vi "Configure Library Classes in Memory for Build.vi"(5 "skip inline classes":string[](array[string]), 7 "target name (My Computer)":string="My Computer", 10 "save VIs? (T)":bool=TRUE, 11 "library name":string="DSF Core.lvlib") -> (0 "error out":errorcluster)   [LabVIEW 2017, in "Build Automation.lvlib"]
uses:
  Build Automation.lvlib
  VI Options.ctl
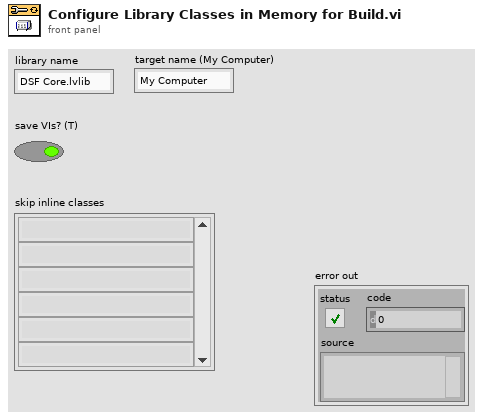
[diagram p1: front panel]
types:
  T1 = typedef "Build Automation.lvlib/VI Options.ctl" = cluster{"Inline":bool, "Is Reentrant":bool, "Reentrancy Type":enum16{"Share clones between instances", "Preallocate clone for each instance"}, "Enable Debugging":bool}
  T2 = cluster{"Status Message":refnum<data-value>, "Progress":refnum<data-value>, "Stop":refnum<data-value>}
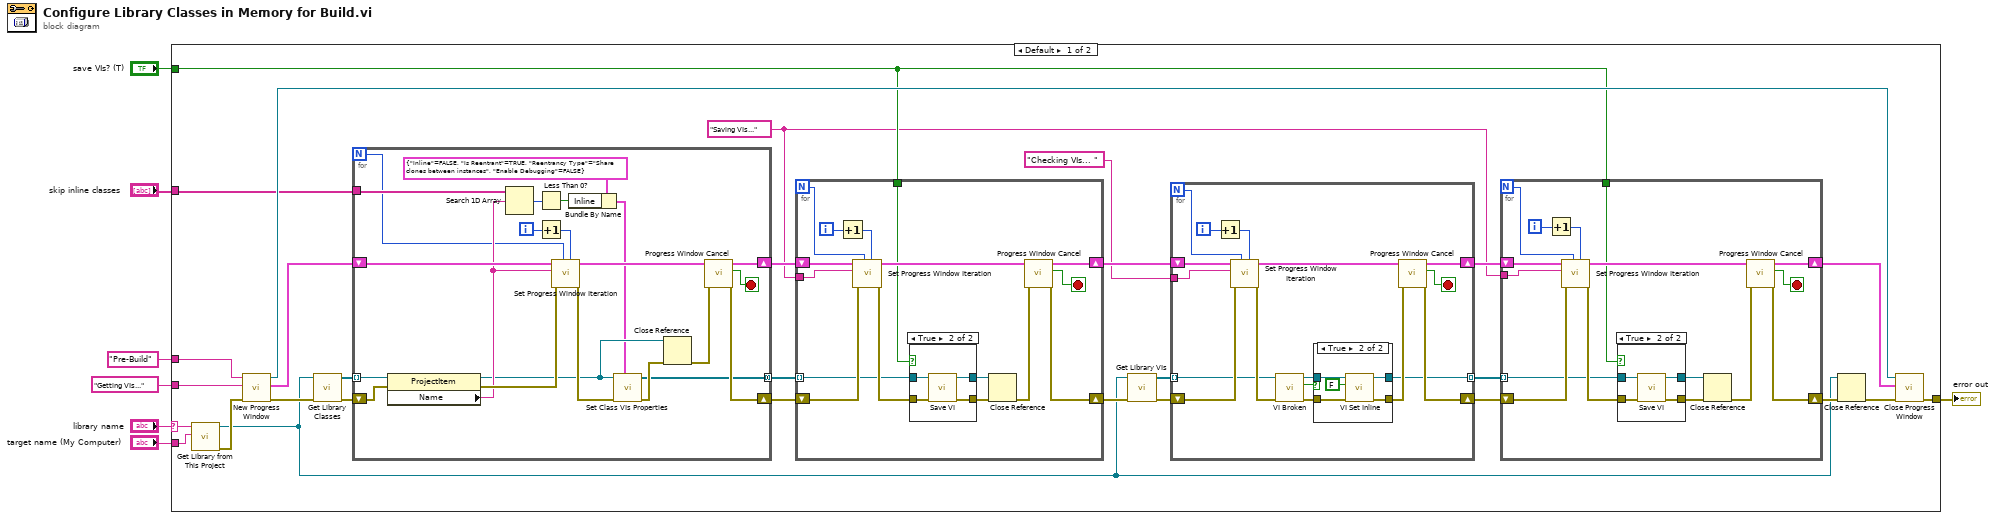
[diagram p0: block diagram]
diagram:
  n1 = case shown="Default" "library name" {
    selector: "library name" -> [w31 _]
    tunnel: [w35 _] -> w7
    tunnel: "save VIs? (T)" -> [w16 _]
    tunnel: "target name (My Computer)" -> [w29 _]
    tunnel: "skip inline classes" -> [w27 _]
    tunnel: "Getting VIs..." ("Initial Message") -> [w12 _]
    tunnel: "Pre-Build" ("WindowTitle") -> [w11 _]
    frame Default {
      w9 = "Saving VIs..." ("Status Message")
      n2 = call "Get Library from This Project.vi"("Target Name (My Computer)"=w29, "Library Name"=w31) -> ("error out"=w30:errorcluster, "Library Refnum"=w10:refnum<vi>)  [unwired: 8 in]
      n3 = call "New Progress Window.vi"("error in (no error)"=w30, "Initial Message"=w12, "Window Title"=w11) -> ("error out"=w22:errorcluster, "DVRs"=w21:T2, "VI refnum"=w36:refnum<vi>)  [unwired: 6 in]
      n4 = call "Get Library Classes.vi"("error in (no error)"=w22, "library ref"=w10) -> ("error out"=w28:errorcluster, "class refs"=w20:refnum<vi>[])  [unwired: 7 in, 1 out]
      n5 = for {
        N -> [w37]
        tunnel: w20 -> [w58] mode=indexing
        shift-right: [w53] -> w19
        shift-left: w28 -> [w57]
        shift-right: [w52] -> w18
        shift-left: w21 -> [w54]
        tunnel: w27 -> [w56]
        tunnel: [w41] -> w17 mode=concatenating
        i -> [w47]
        stop <- w51 stop-if-true
        n6 = property class="ProjectItem"(reference=w58, error in=w57) -> (reference out=w42:refnum<vi>, error out=w49:errorcluster, "Name"=w48:string)
        n7 = Search 1D Array(1D array=w56, element=w48) -> (index of element=w55:i32)  [unwired: 1 in]
        n8 = Less Than 0?(x=w55) -> (x < 0?=w40:bool)
        n9 = Increment(x=w47) -> (x+1=w46:i32)
        n10 = call "Set Progress Window Iteration.vi"("current iteration"=w46, "total iterations"=w37, "error in (no error)"=w49, "Status Message"=w48, "DVRs in"=w54) -> ("error out"=w43:errorcluster, "DVRs out"=w50:T2)  [unwired: 5 in]
        n11 = Bundle By Name(cluster=T1 {"Inline"=FALSE, "Is Reentrant"=TRUE, "Reentrancy Type"=enum."Share clones between instances", "Enable Debugging"=FALSE} ("f"), "Inline"=w40) -> (w38:T1)
        n12 = call "Set Class VIs Properties.vi"("VI Options"=w38, "error in (no error)"=w43, "class ref"=w42) -> ("error out"=w44:errorcluster, "class vi refs"=w41:refnum<vi>[])  [unwired: 7 in]
        n13 = Close Reference(reference=w42, error in (no error)=w44) -> (error out=w45:errorcluster)
        n14 = call "Progress Window Cancel.vi"("error in (no error)"=w45, "DVRs in"=w50) -> ("error out"=w53:errorcluster, "cancelled"=w51:bool, "DVRs out"=w52:T2)  [unwired: 7 in]
      }
      n15 = for {
        N -> [w60]
        shift-right: [w72] -> w14
        shift-left: w18 -> [w71]
        shift-right: [w68] -> w15
        shift-left: w19 -> [w69]
        tunnel: w16 -> [w65]
        tunnel: w17 -> [w64] mode=indexing
        tunnel: w9 -> [w59]
        i -> [w74]
        stop <- w73 stop-if-true
        n16 = Increment(x=w74) -> (x+1=w67:i32)
        n17 = call "Set Progress Window Iteration.vi"("current iteration"=w67, "total iterations"=w60, "error in (no error)"=w69, "Status Message"=w59, "DVRs in"=w71) -> ("error out"=w66:errorcluster, "DVRs out"=w70:T2)  [unwired: 5 in]
        n18 = case shown="True" w65 {
          tunnel: w66 -> [w76 w80]
          tunnel: [w75 w79] -> w63
          tunnel: [w76 w78] -> w62
          tunnel: w64 -> [w75 w77]
          frame False {
          }
          frame True {
            n19 = call "Save VI.vi"("error in (no error)"=w80, "vi ref in"=w77) -> ("error out"=w78:errorcluster, "vi ref out"=w79:refnum<vi>)  [unwired: 8 in]
          }
        }
        n20 = Close Reference(reference=w63, error in (no error)=w62) -> (error out=w61:errorcluster)
        n21 = call "Progress Window Cancel.vi"("error in (no error)"=w61, "DVRs in"=w70) -> ("error out"=w68:errorcluster, "cancelled"=w73:bool, "DVRs out"=w72:T2)  [unwired: 7 in]
      }
      n22 = call "Get Library VIs.vi"("error in (no error)"=w15, "library ref"=w10) -> ("error out"=w23:errorcluster, "vi refs"=w13:refnum<vi>[])  [unwired: 8 in]
      n23 = for {
        N -> [w82]
        tunnel: w13 -> [w88] mode=indexing
        shift-right: [w95] -> w26
        shift-left: w14 -> [w94]
        shift-right: [w91] -> w24
        shift-left: w23 -> [w92]
        tunnel: [w83] -> w25 mode=indexing
        tunnel: "Checking VIs... " ("Status Message") -> [w81]
        i -> [w97]
        stop <- w96 stop-if-true
        n24 = Increment(x=w97) -> (x+1=w90:i32)
        n25 = call "Set Progress Window Iteration.vi"("current iteration"=w90, "total iterations"=w82, "error in (no error)"=w92, "Status Message"=w81, "DVRs in"=w94) -> ("error out"=w89:errorcluster, "DVRs out"=w93:T2)  [unwired: 5 in]
        n26 = call "VI Broken.vi"("error in (no error)"=w89, "vi ref in"=w88) -> ("error out"=w86:errorcluster, "broken?"=w85:bool, "vi ref out"=w87:refnum<vi>)  [unwired: 7 in]
        n27 = case shown="True" w85 {
          tunnel: [w99 w104] -> w83
          tunnel: [w98 w103] -> w84
          tunnel: w86 -> [w98 w102]
          tunnel: w87 -> [w99 w100]
          frame False {
          }
          frame True {
            n28 = call "VI Set Inline.vi"("error in (no error)"=w102, "Inline VI"=FALSE, "vi ref in"=w100) -> ("error out"=w103:errorcluster, "vi ref out"=w104:refnum<vi>)  [unwired: 7 in]
          }
        }
        n29 = call "Progress Window Cancel.vi"("error in (no error)"=w84, "DVRs in"=w93) -> ("error out"=w91:errorcluster, "cancelled"=w96:bool, "DVRs out"=w95:T2)  [unwired: 7 in]
      }
      n30 = for {
        N -> [w106]
        tunnel: w25 -> [w108] mode=indexing
        shift-right: [w118] -> w34
        shift-left: w26 -> [w117]
        shift-right: [w114] -> w33
        shift-left: w24 -> [w115]
        tunnel: w16 -> [w107]
        tunnel: w9 -> [w105]
        i -> [w120]
        stop <- w119 stop-if-true
        n31 = Increment(x=w120) -> (x+1=w113:i32)
        n32 = call "Set Progress Window Iteration.vi"("current iteration"=w113, "total iterations"=w106, "error in (no error)"=w115, "Status Message"=w105, "DVRs in"=w117) -> ("error out"=w112:errorcluster, "DVRs out"=w116:T2)  [unwired: 5 in]
        n33 = case shown="True" w107 {
          tunnel: w112 -> [w121 w126]
          tunnel: [w122 w125] -> w111
          tunnel: [w121 w124] -> w110
          tunnel: w108 -> [w122 w123]
          frame False {
          }
          frame True {
            n34 = call "Save VI.vi"("error in (no error)"=w126, "vi ref in"=w123) -> ("error out"=w124:errorcluster, "vi ref out"=w125:refnum<vi>)  [unwired: 8 in]
          }
        }
        n35 = Close Reference(reference=w111, error in (no error)=w110) -> (error out=w109:errorcluster)
        n36 = call "Progress Window Cancel.vi"("error in (no error)"=w109, "DVRs in"=w116) -> ("error out"=w114:errorcluster, "cancelled"=w119:bool, "DVRs out"=w118:T2)  [unwired: 7 in]
      }
      n37 = Close Reference(reference=w10, error in (no error)=w33) -> (error out=w32:errorcluster)
      n38 = call "Close Progress Window.vi"("error in (no error)"=w32, "DVRs in"=w34, "VI refnum"=w36) -> ("error out"=w35:errorcluster)  [unwired: 8 in]
    }
    frame "" {
    }
  }
  "error out" <- w7
